vi "Set Config Version.vi"(8 "error in (no error)":errorcluster, 10 "Config Version":string, 11 "VolatusConfig in":refnum<class "VolatusConfig.lvclass">) -> (0 "error out":errorcluster, 3 "VolatusConfig out":refnum<class "VolatusConfig.lvclass">)   [LabVIEW 2020, in "VolatusConfig.lvlib" / "VolatusConfig.lvclass"]
uses:
  VolatusConfig.lvclass
  VolatusConfig.lvclass/VolatusConfig.ctl
  lv-cdm/CDM-Config/Config Element/Config Element.lvclass
  Meta Name.ctl
  VolatusConfig.lvlib
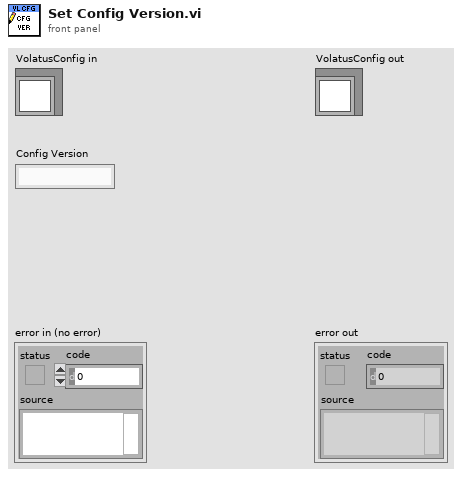
[diagram p1: front panel]
types:
  T1 = typedef "VolatusConfig.lvlib/Meta Name.ctl" = enum16{"VL_Type", "VL_Node_IP", "VL_Node_Type", "VL_Task_Type", "VL_Group_Type", "VL_Channel_Type", "VL_Channel_DataType", "VL_Config_Version", "VL_Overlay_Type"}
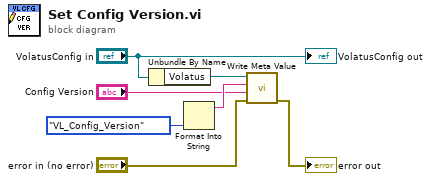
[diagram p0: block diagram]
diagram:
  n1 = Unbundle By Name("VolatusConfig in") -> ("Volatus"=w4:refnum<class "Config Element.lvclass">)
  n2 = Format Into String(Meta_Name."VL_Config_Version" ("Meta Name")) -> (resulting string=w5:string)  [unwired: 3 in, 1 out]
  n3 = call "Write Meta Value.vi"("error in (no error)"="error in (no error)", "Meta Value"="Config Version", "Meta Name"=w5, "Config Element in"=w4) -> ("error out"=→"error out":errorcluster)  [unwired: 6 in, 1 out]
  "VolatusConfig out" <- "VolatusConfig in"
